vi "Write cav_len.vi"(8 "error in (no error)":errorcluster, 10 "cav_len":dbl, 11 "CRDS Cell in":refnum<class "CRDS Cell.lvclass">=refnum) -> (0 "error out":errorcluster, 3 "CRDS Cell out":refnum<class "CRDS Cell.lvclass">)   [LabVIEW 2012]
uses:
  General/Atmospheric/Atmospheric Constants.vi
  General/Atmospheric/Atmospheric Library.lvlib
  CRDS Cell.lvclass
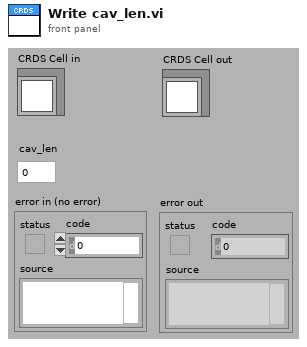
[diagram p1: front panel]
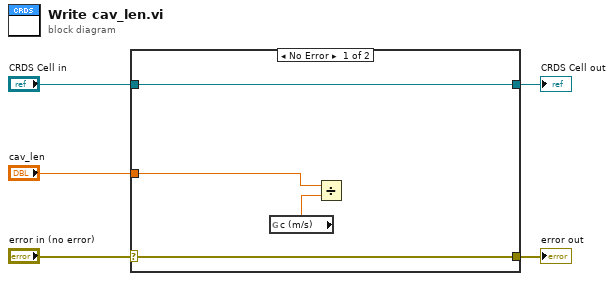
[diagram p0: block diagram]
diagram:
  n1 = case shown="No Error" "error in (no error)" {
    selector: "error in (no error)" -> [w9 w10]
    tunnel: [w9 w10] -> w4
    tunnel: [w6 w11] -> w2
    tunnel: "CRDS Cell in" -> [w6 w11]
    tunnel: "cav_len" -> [w8 _]
    frame No Error {
      n2 = global read "Atmospheric Constants.vi" "c (m/s)"() -> (w7:dbl)
      n3 = Divide(x=w8, y=w7) -> ()  [unwired: 1 out]
    }
    frame Error {
    }
  }
  "error out" <- w4
  "CRDS Cell out" <- w2
